vi "GetSubversionRevision.vi"(11 "File Path Control":path caption="File Path Control (leave blank to use Constants_Global value of EnFlo SW Folder)") -> (0 "This Folder's Last Changed Date":string, 1 "This Folder's Last Revision":string, 2 "LocalModifications":string, 3 "OverallRevision":string, 4 "standard error":string, 5 "standard output":string)   [LabVIEW 2011]
doc: "This VI uses the system's installed svn (subversion) software to return the revision number of the selected folder. Leaving the selected folder blank will use the global value of \"EnFlo SW Folder\".\nThe \"Overall Revision\" is the highest revision number in the entire hierarchy, recursing upwards as well as downwards- in other words, the revision which was checked out. The \"This Folder\" data is specific to the last changes to the selected folder."
uses:
  Anemometry Sub Vis/Globals/Constants_global.vi
panel:
  out "This Folder Last Committed By":string
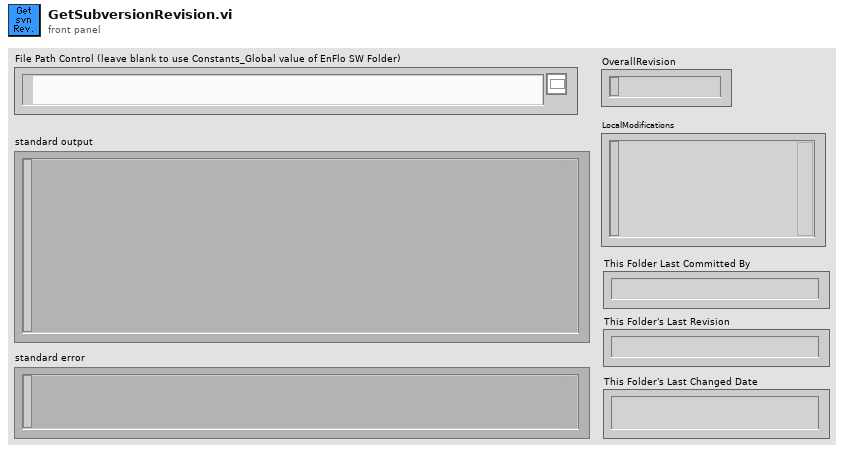
[diagram p1: front panel]
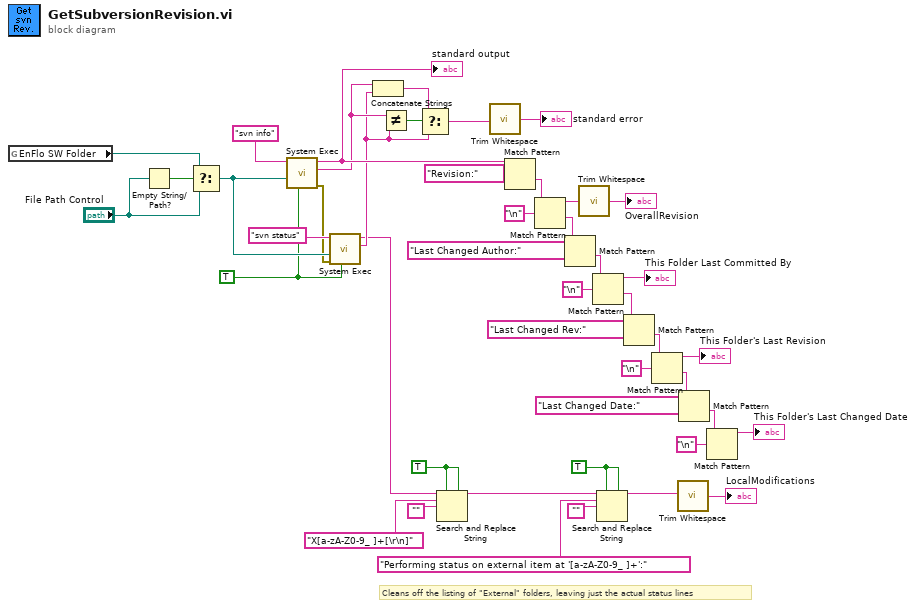
[diagram p0: block diagram]
diagram:
  w5 = TRUE ("replace all? (F)")
  w8 = TRUE ("replace all? (F)")
  w19 = TRUE ("run minimized? (F)")
  # "Cleans off the listing of \"External\" folders, leaving just the actual status lines"
  n1 = global read "Constants_global.vi" "EnFlo SW Folder"() -> (w42:path)
  n2 = Empty String/Path?(string/path="File Path Control") -> (empty?=w44:bool)
  n3 = Select(t=w42, s=w44, f="File Path Control") -> (s? t:f=w21:path)
  n4 = call <vilib>:"System Exec.vi"("run minimized? (F)"=w19, "working directory"=w21, "command line"="svn info") -> ("error out"=w18:errorcluster, "standard error"=w15:string, "standard output"=w41:string)  [unwired: 5 in, 1 out]
  "standard output" <- w41
  n5 = call <vilib>:"System Exec.vi"("run minimized? (F)"=w19, "error in (no error)"=w18, "working directory"=w21, "command line"="svn status") -> ("standard error"=w11:string, "standard output"=w7:string)  [unwired: 4 in, 2 out]
  n6 = Concatenate Strings(w15, w11) -> (w13:string)
  n7 = Not Equal?(x=w15, y=w11) -> (x != y?=w14:bool)
  n8 = Select(t=w13, s=w14, f=w11) -> (s? t:f=w12:string)
  n9 = Search and Replace String(replace all?=w8, multiline?=w8, input string=w7, search string="X[a-zA-Z0-9_ ]+[\r\n]", replace string="") -> (result string=w3:string)  [unwired: 3 in, 3 out]
  n10 = call <vilib>:"Trim Whitespace.vi"("string"=w12) -> ("trimmed string"=→"standard error":string)  [unwired: 1 in]
  n11 = Match Pattern(string=w41, regular expression="Revision:") -> (after substring=w39:string)  [unwired: 1 in, 3 out]
  n12 = Match Pattern(string=w39, regular expression="\n") -> (before substring=w37:string, after substring=w36:string)  [unwired: 1 in, 2 out]
  n13 = Match Pattern(string=w36, regular expression="Last Changed Author:") -> (after substring=w33:string)  [unwired: 1 in, 3 out]
  n14 = call <vilib>:"Trim Whitespace.vi"("string"=w37) -> ("trimmed string"=→"OverallRevision":string)  [unwired: 1 in]
  n15 = Match Pattern(string=w33, regular expression="\n") -> (before substring=→"This Folder Last Committed By":string, after substring=w29:string)  [unwired: 1 in, 2 out]
  n16 = Search and Replace String(replace all?=w5, multiline?=w5, input string=w3, search string="Performing status on external item at '[a-zA-Z0-9_ ]+':", replace string="") -> (result string=w2:string)  [unwired: 3 in, 3 out]
  n17 = Match Pattern(string=w29, regular expression="Last Changed Rev:") -> (after substring=w31:string)  [unwired: 1 in, 3 out]
  n18 = Match Pattern(string=w31, regular expression="\n") -> (before substring=→"This Folder's Last Revision":string, after substring=w24:string)  [unwired: 1 in, 2 out]
  n19 = call <vilib>:"Trim Whitespace.vi"("string"=w2) -> ("trimmed string"=→"LocalModifications":string)  [unwired: 1 in]
  n20 = Match Pattern(string=w24, regular expression="Last Changed Date:") -> (after substring=w25:string)  [unwired: 1 in, 3 out]
  n21 = Match Pattern(string=w25, regular expression="\n") -> (before substring=→"This Folder's Last Changed Date":string)  [unwired: 1 in, 3 out]
